vi "PhoenixPro_Device_RefNumRegistrySet.vi"(8 "error in (no error)":errorcluster, 9 "Test Mode Only":bool, 10 "refnum name":string="Talon", 11 "DeviceReference":T1) -> (0 "error out":errorcluster, 3 "data":T1)   [LabVIEW 2020]
uses:
  DeviceReference.ctl
  <vilib>/Rock Robotics/WPI/Utilities/Refnum Registry Operation.ctl
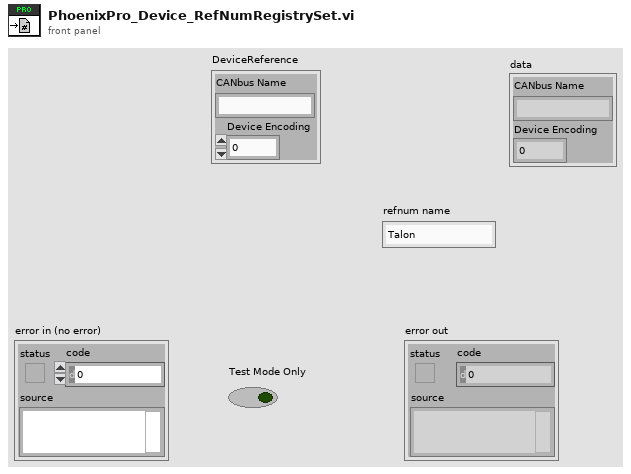
[diagram p1: front panel]
types:
  T1 = typedef "DeviceReference.ctl" = cluster{"CANbus Name":string, "Device Encoding":u32}
  T2 = typedef "Refnum Registry Operation.ctl" = enum16{"set", "get", "delete", "get all names", "read name"}
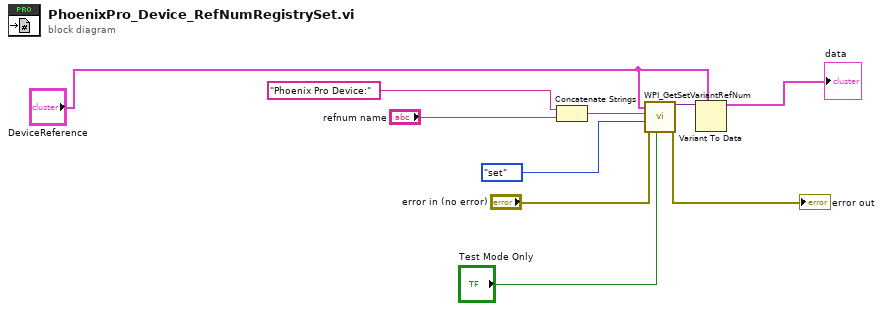
[diagram p0: block diagram]
diagram:
  n1 = Concatenate Strings("Phoenix Pro Device:", "refnum name") -> (w10:string)
  n2 = call <vilib>:"WPI_GetSetVariantRefNum.vi"("Test Mode Only"="Test Mode Only", "error in (no error)"="error in (no error)", "Operation"=Refnum_Registry_Operation."set" ("menu"), "refnum name"=w10, "DevRef"="DeviceReference") -> ("error out"=→"error out":errorcluster, "DevRef"=w8:variant)  [unwired: 4 in, 1 out]
  n3 = Variant To Data(type="DeviceReference", Variant=w8) -> (data=→"data":T1)  [unwired: 1 in, 1 out]
